vi "Write.vi"   [LabVIEW 2011, in "LVH-Adept.lvlib"]
uses:
  <vilib>/LabVIEW Hacker/Adept/LVH-Adept.lvlib
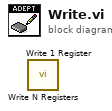
[diagram p0: block diagram]
diagram:
  n1 = call <vilib>:"Write N Registers.vi"() -> ()  [unwired: 10 in, 2 out]
  n2 = call <vilib>:"Write 1 Register.vi"() -> ()  [unwired: 10 in, 2 out]
